vi "mqttKeepAliveWrite.vi"(0 "mqtt in":refnum<class "mqtt.lvclass">, 5 "keepAlive(sec)":u16=60, 11 "error in (no error)":errorcluster) -> (4 "mqtt out":refnum<class "mqtt.lvclass">, 15 "error out":errorcluster)   [LabVIEW 2018, in "labview-mqtt.lvlib" / "mqtt.lvclass"]
uses:
  mqtt.lvclass
  mqtt.lvclass/mqtt.ctl
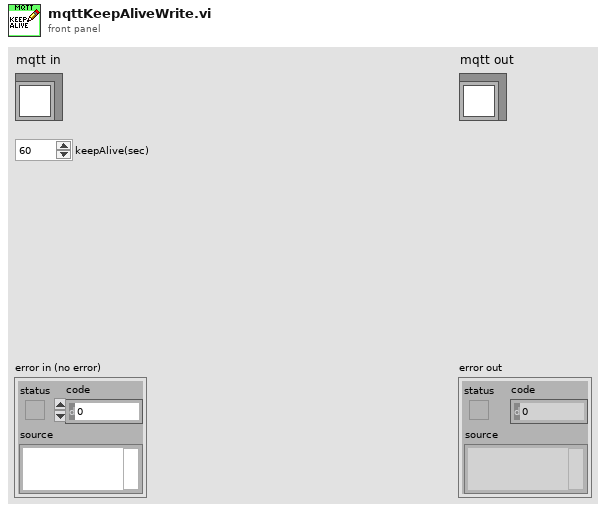
[diagram p1: front panel]
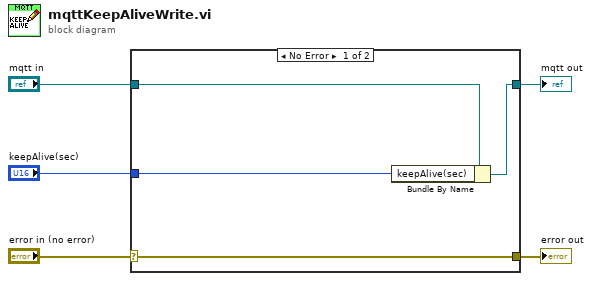
[diagram p0: block diagram]
diagram:
  n1 = case shown="No Error" "error in (no error)" {
    selector: "error in (no error)" -> [w9 w10]
    tunnel: [w9 w10] -> w4
    tunnel: [w7 w11] -> w2
    tunnel: "mqtt in" -> [w8 w11]
    tunnel: "keepAlive(sec)" -> [w6 _]
    frame No Error {
      n2 = Bundle By Name(cluster=w8, "keepAlive(sec)"=w6) -> (w7:refnum<class "mqtt.lvclass">)
    }
    frame Error {
    }
  }
  "error out" <- w4
  "mqtt out" <- w2
